vi "Flush Data.vi"(0 "UART Driver in":refnum<class "UART Driver.lvclass">, 5 "Flush Options":T1=enum."Tx & Rx", 11 "error in":errorcluster) -> (4 "UART Driver out":refnum<class "UART Driver.lvclass">, 15 "error out":errorcluster)   [LabVIEW 2012, in "UART_Host_Driver.lvlib" / "UART Driver.lvclass"]
uses:
  UART Driver.lvclass
  Typedefs/Flush Options.ctl
  Typedefs/FPGA VI Reference.ctl
  UART Driver.lvclass/UART Driver.ctl
  <vilib>/Utility/error.llb/Error Cluster From Error Code.vi
  <vilib>/rvi/interface/nirviMethod/nirviMethod.xnode
  UART_Host_Driver.lvlib
  <vilib>/rvi/errors/niLvFpgaMergeErrorWithErrorCode.vi
  <vilib>/FPGAPlugInAG/Dynamic/niLvFpga_StopFifo_Dynamic.vi
  <vilib>/FPGAPlugInAG/Dynamic/niLvFpga_StartFifo_Dynamic.vi
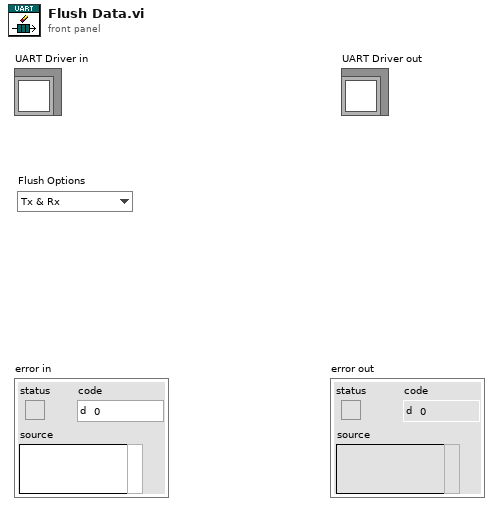
[diagram p1: front panel]
types:
  T1 = typedef "UART_Host_Driver.lvlib/Flush Options.ctl" = enum16{"Tx", "Rx", "Tx & Rx"}
  T2 = typedef "UART_Host_Driver.lvlib/FPGA VI Reference.ctl" = refnum<k20>
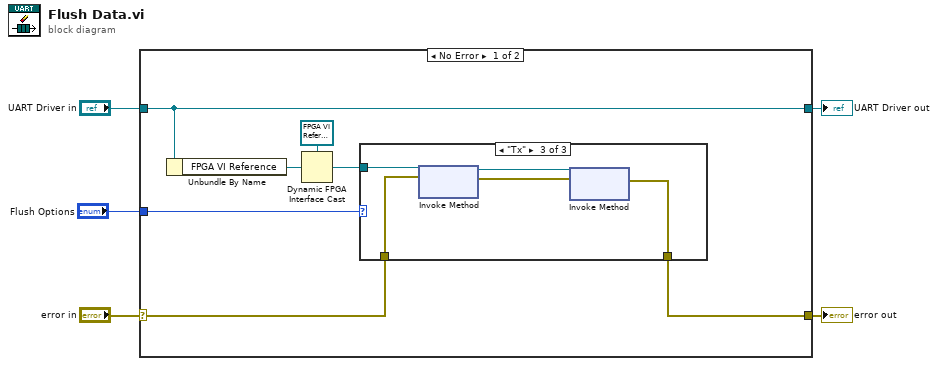
[diagram p0: block diagram]
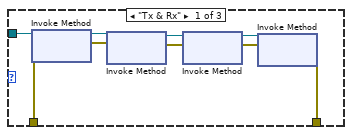
[diagram p2: hidden frame]
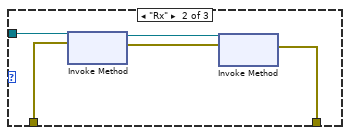
[diagram p3: hidden frame]
diagram:
  n1 = case shown="No Error" "error in" {
    selector: "error in" -> [w8 w33]
    tunnel: [w6 w33] -> w4
    tunnel: [w12 w32] -> w2
    tunnel: "UART Driver in" -> [w12 w32]
    tunnel: "Flush Options" -> [w7 _]
    frame No Error {
      n2 = Unbundle By Name(w12) -> ("FPGA VI Reference"=w11:refnum<k20>)
      n3 = Dynamic FPGA Interface Cast(Session In=T2 refnum ("FPGA VI Reference"), Type=w11) -> (Session Out=w9:T2)
      n4 = case shown="\"Tx\"" w7 {
        tunnel: w9 -> [w21 w25 w30]
        tunnel: w8 -> [w20 w24 w29]
        tunnel: [w13 w26 w31] -> w6
        frame "Tx & Rx" {
          n5 = xnode "Invoke Method"("FPGA VI Reference In"=w21, "error in"=w20) -> ("FPGA VI Reference Out"=w19:T2, "error out"=w18:errorcluster)
          n6 = xnode "Invoke Method"("FPGA VI Reference In"=w19, "error in"=w18) -> ("FPGA VI Reference Out"=w16:T2, "error out"=w15:errorcluster)
          n7 = xnode "Invoke Method"("FPGA VI Reference In"=w16, "error in"=w15) -> ("FPGA VI Reference Out"=w14:T2, "error out"=w17:errorcluster)
          n8 = xnode "Invoke Method"("FPGA VI Reference In"=w14, "error in"=w17) -> ("error out"=w13:errorcluster)  [unwired: 1 out]
        }
        frame "Rx" {
          n9 = xnode "Invoke Method"("FPGA VI Reference In"=w25, "error in"=w24) -> ("FPGA VI Reference Out"=w23:T2, "error out"=w22:errorcluster)
          n10 = xnode "Invoke Method"("FPGA VI Reference In"=w23, "error in"=w22) -> ("error out"=w26:errorcluster)  [unwired: 1 out]
        }
        frame "Tx" {
          n11 = xnode "Invoke Method"("FPGA VI Reference In"=w30, "error in"=w29) -> ("FPGA VI Reference Out"=w28:T2, "error out"=w27:errorcluster)
          n12 = xnode "Invoke Method"("FPGA VI Reference In"=w28, "error in"=w27) -> ("error out"=w31:errorcluster)  [unwired: 1 out]
        }
      }
    }
    frame Error {
    }
  }
  "error out" <- w4
  "UART Driver out" <- w2
